vi "Servicio Hardware.vi"(11 "Caracter Servicio":string="T") -> ()   [LabVIEW 2020, in "Hardware.lvlib"]
uses:
  Hardware.lvlib
  <vilib>/Instr/_visa.llb/VISA Configure Serial Port (Instr).vi
panel:
  out "error out":errorcluster
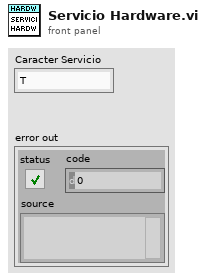
[diagram p1: front panel]
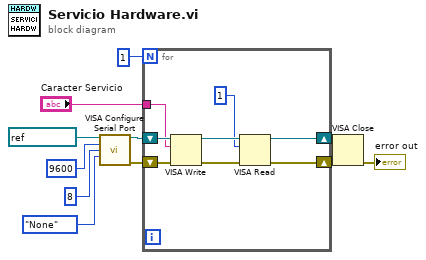
[diagram p0: block diagram]
diagram:
  n1 = call-poly "VISA Configure Serial Port"("VISA resource name"=refnum<visa-resource-name> "COM10" ("Serial"), "baud rate (9600)"=u32 9600, "data bits (8)"=u16 8, "parity (0:none)"=enum16{"None", "Odd", "Even", "Mark", "Space"}."None") -> ("VISA resource name out"=w5:refnum<visa-resource-name>, "error out"=w4:errorcluster)  [unwired: 10 in]
  n2 = for {
    N: 1 -> [_]
    shift-right: [w19] -> w11
    shift-left: w5 -> [w17]
    shift-right: [w18] -> w10
    shift-left: w4 -> [w16]
    tunnel: "Caracter Servicio" -> [w12]
    n3 = VISA Write(VISA resource name=w17, write buffer=w12, error in (no error)=w16) -> (VISA resource name out=w15:refnum<visa-resource-name>, error out=w14:errorcluster)  [unwired: 1 out]
    n4 = VISA Read(VISA resource name=w15, byte count=u32 1, error in (no error)=w14) -> (VISA resource name out=w19:refnum<visa-resource-name>, error out=w18:errorcluster)  [unwired: 2 out]
  }
  n5 = VISA Close(VISA resource name=w11, error in (no error)=w10) -> (error out=→"error out":errorcluster)
